vi "measure att. peaks.vi"(4 "Label offsets":cluster{"x":dbl, "y":dbl}, 6 "Peak annot. color":u32(colorbox), 7 "First anott. index":i32=15, 8 "error in":errorcluster, 9 "Plot":dbl[][](array[numeric]), 10 "crossovers":dbl[](array[numeric]), 11 "XYGraph in":refnum<vi>) -> (0 "error out":errorcluster, 3 "XYGraph out":refnum<vi>)   [LabVIEW 2014]
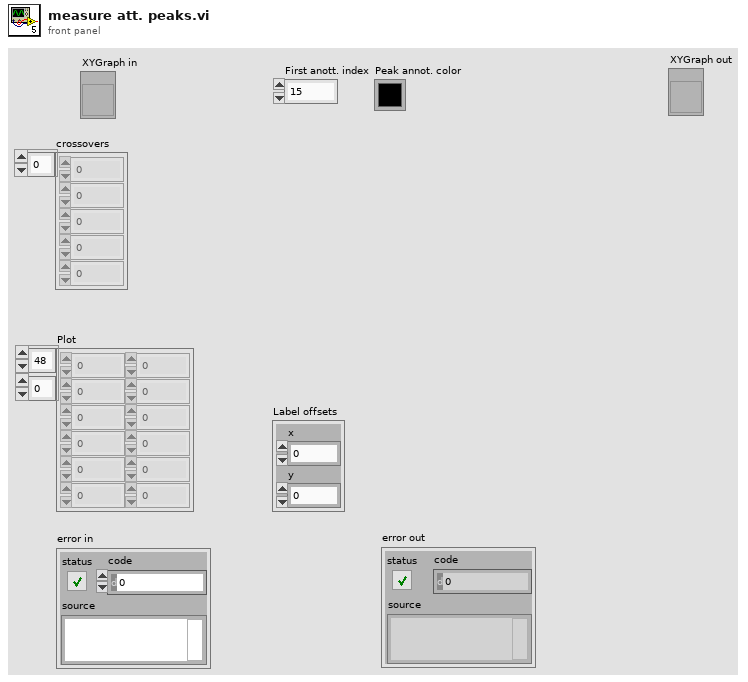
[diagram p1: front panel]
types:
  T1 = typedef "LVAnnotationListTypeDef.ctl" = cluster{"Name":string, "Color":u32, "Style":u8, "Point Style":u8, "Name Visible":bool, "Allow Drag":bool, "Annotation Mode":u32, "Plot":i32, "Index":i32, "Position":cluster{"X":dbl, "Y":dbl}, "X Scale":u32, "Y Scale":u32, "Show Arrow":bool, "Lock Name":bool, "Plot Area":i32, "Label Offset":cluster{"X":dbl, "Y":dbl}}[]
  T2 = cluster{"Name":string, "Color":u32, "Style":u8, "Point Style":u8, "Name Visible":bool, "Allow Drag":bool, "Annotation Mode":u32, "Plot":i32, "Index":i32, "Position":cluster{"X":dbl, "Y":dbl}, "X Scale":u32, "Y Scale":u32, "Show Arrow":bool, "Lock Name":bool, "Plot Area":i32, "Label Offset":cluster{"X":dbl, "Y":dbl}}
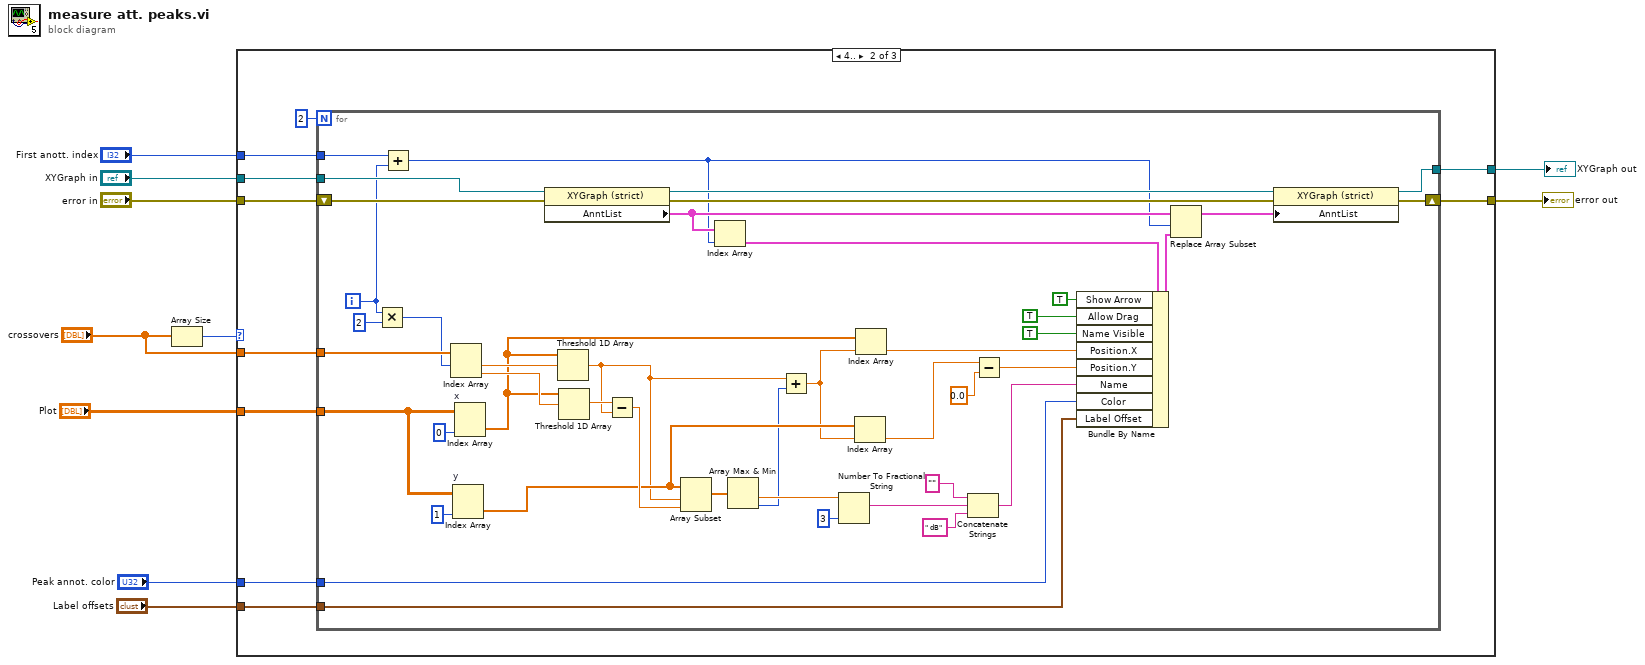
[diagram p0: block diagram]
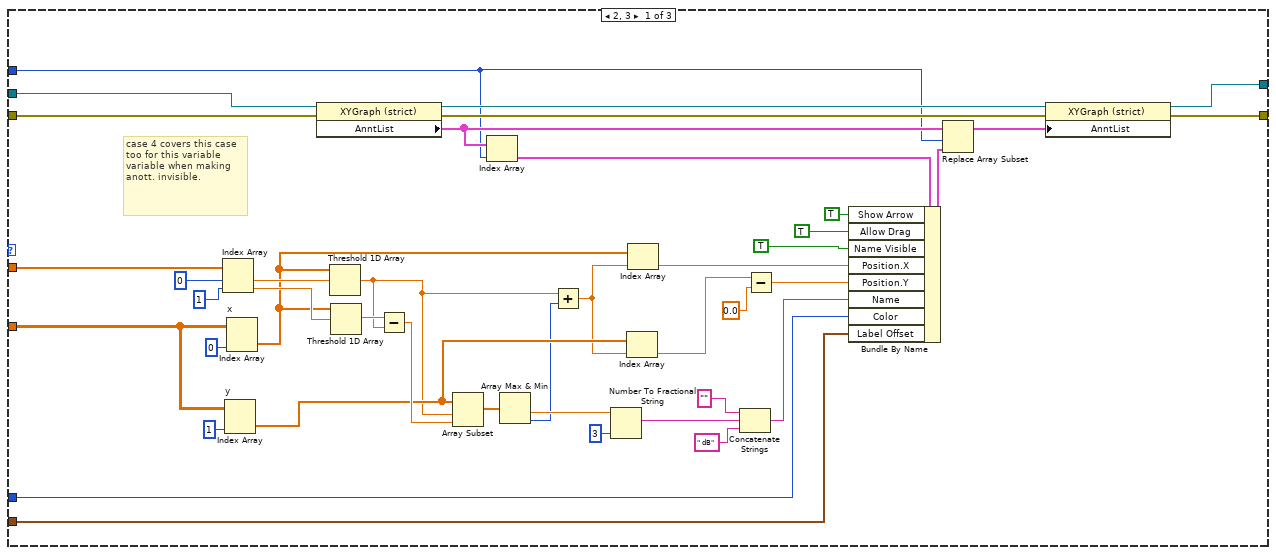
[diagram p2: hidden frame]
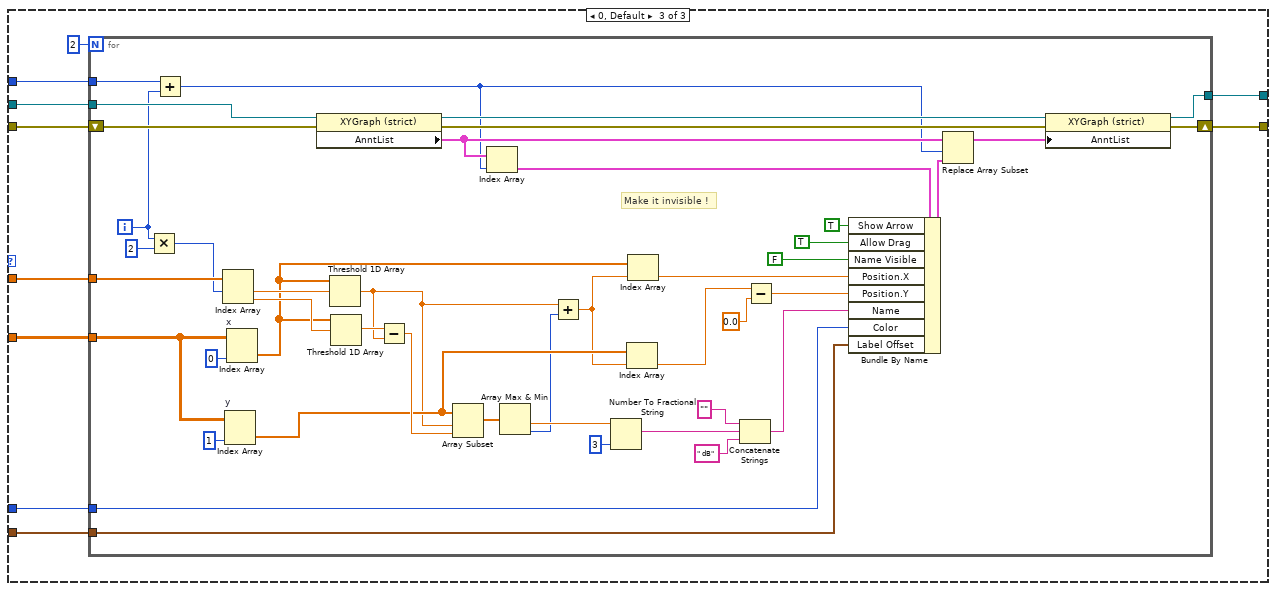
[diagram p3: hidden frame]
diagram:
  n1 = Array Size(array="crossovers") -> (size(s)=w10:i32)
  n2 = case shown="4.." w10 {
    tunnel: "Plot" -> [w48 w61 w115]
    tunnel: "crossovers" -> [w51 w62 w116]
    tunnel: "XYGraph in" -> [w41 w60 w114]
    tunnel: "First anott. index" -> [w20 w59 w113]
    tunnel: "error in" -> [w19 w58 w112]
    tunnel: [w18 w57 w111] -> w4
    tunnel: "Peak annot. color" -> [w13 w55 w109]
    tunnel: [w14 w54 w108] -> w2
    tunnel: "Label offsets" -> [w12 w53 w107]
    frame 2, 3 {
      # "case 4 covers this case too for this variable\nvariable when making anott. invisible."
      n3 = Index Array(array=w51, index #1=0 ("index"), index #2=1 ("index")) -> (element #1=w46:dbl, element #2=w45:dbl)
      n4 = Index Array "y"(array=w48, index (col)=1 ("disabled index (col)")) -> (element=w34:dbl[])  [unwired: 1 in]
      n5 = Index Array "x"(array=w48, index (col)=0 ("disabled index (col)")) -> (element=w32:dbl[])  [unwired: 1 in]
      n6 = property class="XYGraph (strict)"(reference=w41, error in=w19) -> (reference out=w37:refnum<vi>, error out=w31:errorcluster, "AnntList"=w40:T1)
      n7 = Threshold 1D Array(2:w46, 3:w32) -> (0:w15:dbl)  [unwired: 1 in]
      n8 = Threshold 1D Array(2:w45, 3:w32) -> (0:w44:dbl)  [unwired: 1 in]
      n9 = Subtract(x=w44, y=w15) -> (x-y=w43:dbl)
      n10 = Array Subset(array=w34, index=w15, length=w43) -> (w42:dbl[])
      n11 = Index Array(array=w40, index=w20) -> (element=w39:T2)
      n12 = Array Max & Min(array=w42) -> (min value=w30:dbl, min index (indices)=w16:i32)  [unwired: 2 out]
      n13 = Add(x=w15, y=w16) -> (x+y=w17:dbl)
      n14 = Number To Fractional String(number=w30, precision (6)=i16 3) -> (F-format string=w28:string)  [unwired: 2 in]
      n15 = Index Array(array=w34, index=w17) -> (element=w23:dbl)
      n16 = Index Array(array=w32, index=w17) -> (element=w33:dbl)
      n17 = Concatenate Strings("" ("string"), w28, " dB" ("string")) -> (w25:string)
      n18 = Subtract(x=w23, y=0.0) -> (x-y=w22:dbl)
      n19 = Bundle By Name(cluster=w39, "Show Arrow"=TRUE, "Allow Drag"=TRUE, "Name Visible"=TRUE, "Position.X"=w33, "Position.Y"=w22, "Name"=w25, "Color"=w13, "Label Offset"=w12) -> (w38:T2)
      n20 = Replace Array Subset(array=w40, new element=w38, index=w20) -> (w36:T1)
      n21 = property class="XYGraph (strict)"(reference=w37, error in=w31, "AnntList"=w36) -> (reference out=w14:refnum<vi>, error out=w18:errorcluster)
    }
    frame 4.. {
      n22 = for {
        N: 2 -> [_]
        tunnel: w62 -> [w105]
        tunnel: w61 -> [w104]
        tunnel: w60 -> [w97]
        tunnel: w59 -> [w69]
        shift-right: [w76] -> w57
        shift-left: w58 -> [w77]
        tunnel: w55 -> [w66]
        tunnel: [w67] -> w54
        tunnel: w53 -> [w65]
        i -> [w68]
        n23 = Multiply(x=w68, y=2) -> (x*y=w71:i32)
        n24 = Add(x=w69, y=w68) -> (x+y=w70:i32)
        n25 = Index Array(array=w105, index #1=w71) -> (element #1=w102:dbl, element #2=w101:dbl)  [unwired: 1 in]
        n26 = Index Array "y"(array=w104, index (col)=1 ("disabled index (col)")) -> (element=w91:dbl[])  [unwired: 1 in]
        n27 = Index Array "x"(array=w104, index (col)=0 ("disabled index (col)")) -> (element=w89:dbl[])  [unwired: 1 in]
        n28 = property class="XYGraph (strict)"(reference=w97, error in=w77) -> (reference out=w93:refnum<vi>, error out=w88:errorcluster, "AnntList"=w96:T1)
        n29 = Threshold 1D Array(2:w102, 3:w89) -> (0:w73:dbl)  [unwired: 1 in]
        n30 = Threshold 1D Array(2:w101, 3:w89) -> (0:w100:dbl)  [unwired: 1 in]
        n31 = Subtract(x=w100, y=w73) -> (x-y=w99:dbl)
        n32 = Array Subset(array=w91, index=w73, length=w99) -> (w98:dbl[])
        n33 = Index Array(array=w96, index=w70) -> (element=w95:T2)
        n34 = Array Max & Min(array=w98) -> (min value=w87:dbl, min index (indices)=w74:i32)  [unwired: 2 out]
        n35 = Add(x=w73, y=w74) -> (x+y=w75:dbl)
        n36 = Number To Fractional String(number=w87, precision (6)=i16 3) -> (F-format string=w85:string)  [unwired: 2 in]
        n37 = Index Array(array=w91, index=w75) -> (element=w80:dbl)
        n38 = Index Array(array=w89, index=w75) -> (element=w90:dbl)
        n39 = Concatenate Strings("" ("string"), w85, " dB" ("string")) -> (w82:string)
        n40 = Subtract(x=w80, y=0.0) -> (x-y=w79:dbl)
        n41 = Bundle By Name(cluster=w95, "Show Arrow"=TRUE, "Allow Drag"=TRUE, "Name Visible"=TRUE, "Position.X"=w90, "Position.Y"=w79, "Name"=w82, "Color"=w66, "Label Offset"=w65) -> (w94:T2)
        n42 = Replace Array Subset(array=w96, new element=w94, index=w70) -> (w92:T1)
        n43 = property class="XYGraph (strict)"(reference=w93, error in=w88, "AnntList"=w92) -> (reference out=w67:refnum<vi>, error out=w76:errorcluster)
      }
    }
    frame 0, Default {
      n44 = for {
        N: 2 -> [_]
        tunnel: w116 -> [w159]
        tunnel: w115 -> [w158]
        tunnel: w114 -> [w151]
        tunnel: w113 -> [w123]
        shift-right: [w130] -> w111
        shift-left: w112 -> [w131]
        tunnel: w109 -> [w120]
        tunnel: [w121] -> w108
        tunnel: w107 -> [w119]
        i -> [w122]
        # "Make it invisible !"
        n45 = Multiply(x=w122, y=2) -> (x*y=w125:i32)
        n46 = Add(x=w123, y=w122) -> (x+y=w124:i32)
        n47 = Index Array(array=w159, index #1=w125) -> (element #1=w156:dbl, element #2=w155:dbl)  [unwired: 1 in]
        n48 = Index Array "y"(array=w158, index (col)=1 ("disabled index (col)")) -> (element=w145:dbl[])  [unwired: 1 in]
        n49 = Index Array "x"(array=w158, index (col)=0 ("disabled index (col)")) -> (element=w143:dbl[])  [unwired: 1 in]
        n50 = property class="XYGraph (strict)"(reference=w151, error in=w131) -> (reference out=w147:refnum<vi>, error out=w142:errorcluster, "AnntList"=w150:T1)
        n51 = Threshold 1D Array(2:w156, 3:w143) -> (0:w127:dbl)  [unwired: 1 in]
        n52 = Threshold 1D Array(2:w155, 3:w143) -> (0:w154:dbl)  [unwired: 1 in]
        n53 = Subtract(x=w154, y=w127) -> (x-y=w153:dbl)
        n54 = Array Subset(array=w145, index=w127, length=w153) -> (w152:dbl[])
        n55 = Index Array(array=w150, index=w124) -> (element=w149:T2)
        n56 = Array Max & Min(array=w152) -> (min value=w141:dbl, min index (indices)=w128:i32)  [unwired: 2 out]
        n57 = Add(x=w127, y=w128) -> (x+y=w129:dbl)
        n58 = Number To Fractional String(number=w141, precision (6)=i16 3) -> (F-format string=w139:string)  [unwired: 2 in]
        n59 = Index Array(array=w145, index=w129) -> (element=w134:dbl)
        n60 = Index Array(array=w143, index=w129) -> (element=w144:dbl)
        n61 = Concatenate Strings("" ("string"), w139, " dB" ("string")) -> (w136:string)
        n62 = Subtract(x=w134, y=0.0) -> (x-y=w133:dbl)
        n63 = Bundle By Name(cluster=w149, "Show Arrow"=TRUE, "Allow Drag"=TRUE, "Name Visible"=FALSE, "Position.X"=w144, "Position.Y"=w133, "Name"=w136, "Color"=w120, "Label Offset"=w119) -> (w148:T2)
        n64 = Replace Array Subset(array=w150, new element=w148, index=w124) -> (w146:T1)
        n65 = property class="XYGraph (strict)"(reference=w147, error in=w142, "AnntList"=w146) -> (reference out=w121:refnum<vi>, error out=w130:errorcluster)
      }
    }
  }
  "error out" <- w4
  "XYGraph out" <- w2
